vi "Read Config Accessor.vi"(8 "error in (no error)":errorcluster, 11 "LiDAR in":refnum<class "LiDAR.lvclass">) -> (0 "error out":errorcluster, 2 "Configuration":refnum<class "Configuration.lvclass">, 3 "LiDAR out":refnum<class "LiDAR.lvclass">)   [LabVIEW 2018, in "LiDAR.lvlib" / "LiDAR.lvclass"]
uses:
  LiDAR.lvclass
  PPLs/Configuration/Configuration.lvlibp/Configuration.lvclass
  LiDAR.lvclass/LiDAR.ctl
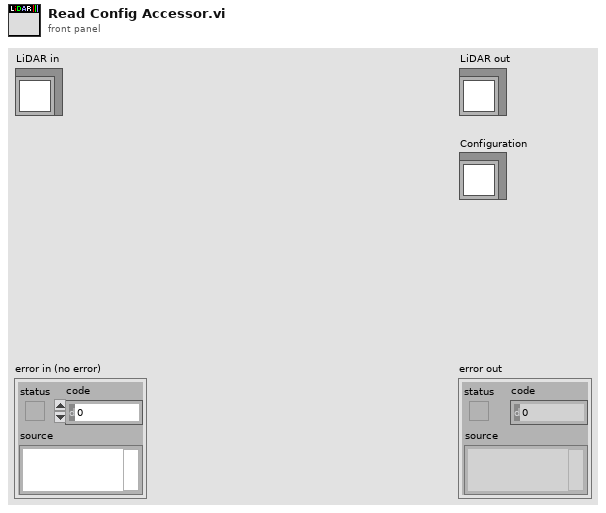
[diagram p1: front panel]
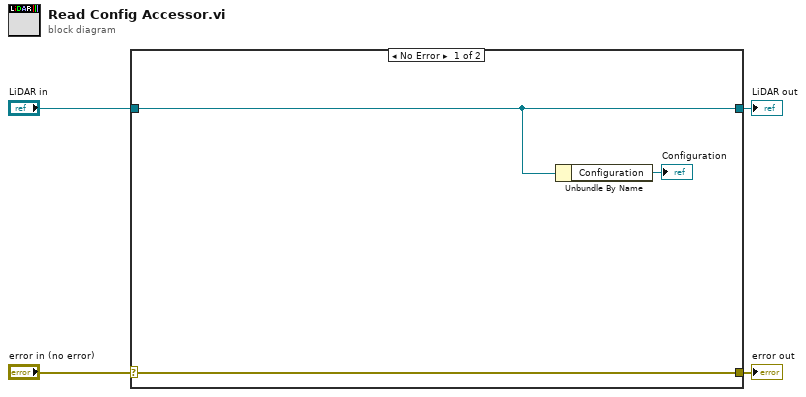
[diagram p0: block diagram]
diagram:
  n1 = case shown="No Error" "error in (no error)" {
    selector: "error in (no error)" -> [w7 w9]
    tunnel: [w7 w9] -> w3
    tunnel: [w6 w8] -> w1
    tunnel: "LiDAR in" -> [w6 w8]
    frame No Error {
      n2 = Unbundle By Name(w6) -> ("Configuration"=→"Configuration":refnum<class "Configuration.lvclass">)
    }
    frame Error {
    }
  }
  "error out" <- w3
  "LiDAR out" <- w1
